vi "Find Setpoint.vi"(8 "error in (no error)":errorcluster, 11 "Settings in":T1 {"Processing Settings"."Test Parameters"."Allowed Tolerance (%) FS" format="%#_4g"; "Acq Settings"."Config Settings"."Simulated Sensor Injection" scale=0.0..100.0}) -> (0 "error out":errorcluster, 3 "Settings out":T1 {"Processing Settings"."Test Parameters"."Allowed Tolerance (%) FS" format="%#_4g"; "Acq Settings"."Config Settings"."Simulated Sensor Injection" scale=0.0..100.0})   [LabVIEW 2026]
uses:
  controls/UI/Settings Cluster.ctl
  controls/UI/Acq Settings.ctl
  Acquisition/Instrument Specifications Configuration.ctl
  Acquisition/Instrument Specifications Cluster Configuration.ctl
  controls/UI/Measurement Role.ctl
  controls/UI/Config Settings.ctl
  Processing/Processing Settings.ctl
  controls/Messaging Payloads/Sensor CoreData.ctl
  controls/Messaging Payloads/Sensor CoreData Cluster.ctl
  controls/UI/Units Enum.ctl
  controls/UI/Signal Enum.ctl
  Processing/Test Parameters.ctl
  Processing/Test Parameters Cluster.ctl
  controls/UI/Test Sequence Context.ctl
  controls/UI/Test Sequence Context Cluster.ctl
  controls/UI/Direction.ctl
  controls/UI/Session Identfiers.ctl
  controls/UI/Test Sequence Settings.ctl
  controls/UI/Test Sequence State.ctl
  controls/UI/Test Sequence Enum.ctl
  controls/Controller/Stimulus Settings.ctl
  controls/Controller/Stimulus Outputs.ctl
  controls/Controller/Stimulus Output.ctl
  controls/Controller/Controller Core Data.ctl
  controls/Controller/Stimulus Output Configuration.ctl
  controls/Controller/Stimulus Role.ctl
  Settings/Settings.lvlib
  Acquisition/Acquisition.lvlib
  Processing/Processing_Engine.lvlib
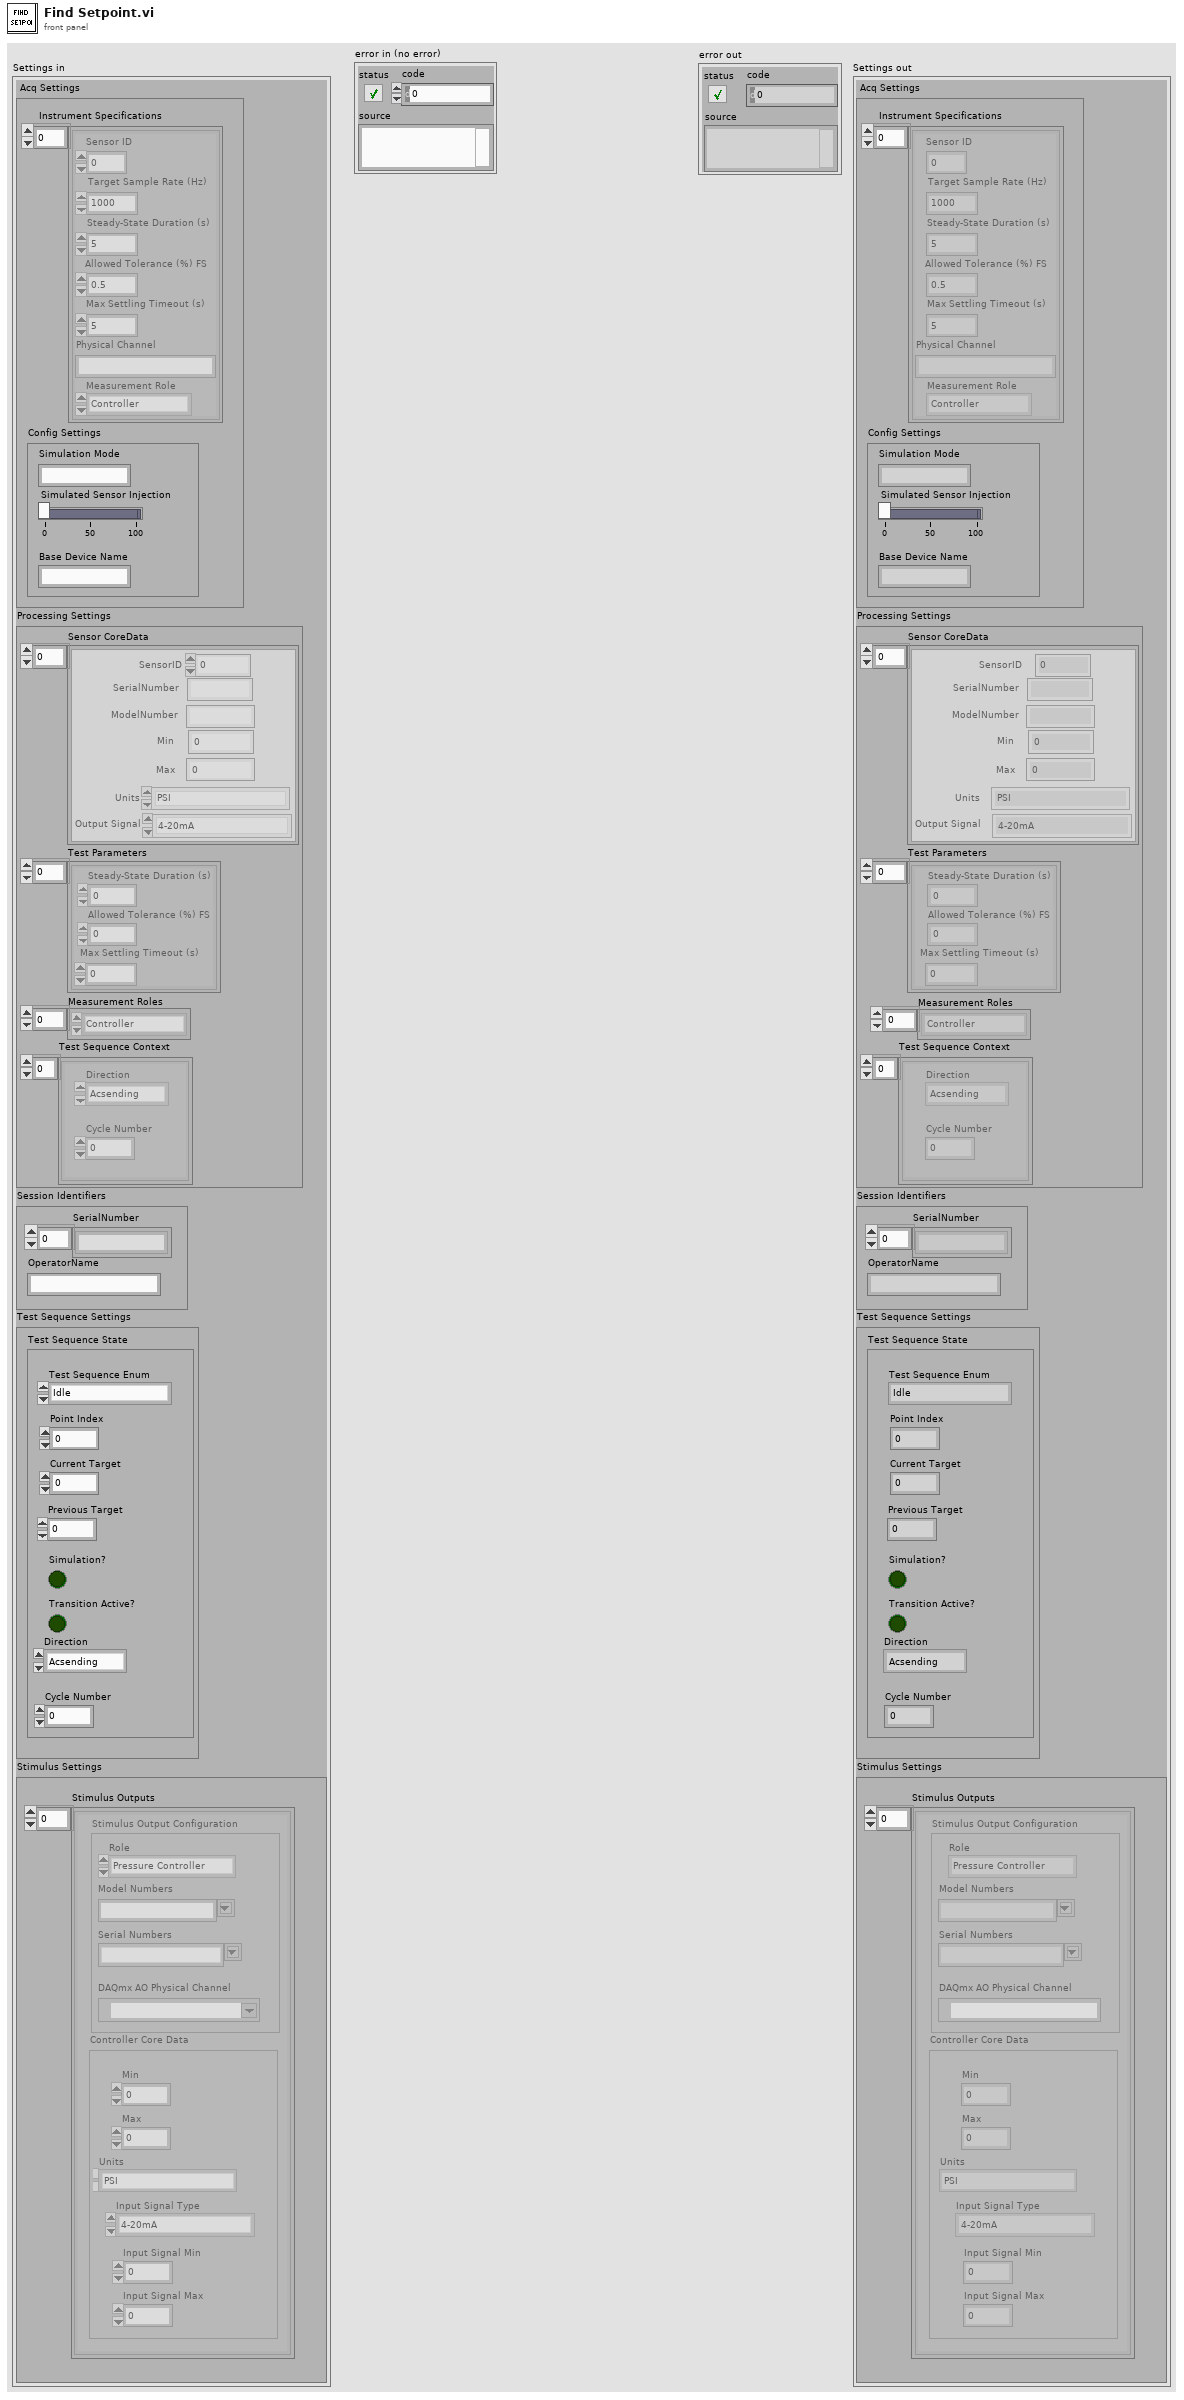
[diagram p1: front panel]
types:
  T1 = typedef "Settings Cluster.ctl" = cluster{"Acq Settings":T2, "Processing Settings":T7, "Session Identifiers":T17, "Test Sequence Settings":T18, "Stimulus Settings":T21}
  T2 = typedef "Acq Settings.ctl" = cluster{"Instrument Specifications":T3, "Config Settings":T6}
  T3 = typedef "Acquisition.lvlib/Instrument Specifications Configuration.ctl" = T4[]
  T4 = typedef "Acquisition.lvlib/Instrument Specifications Cluster Configuration.ctl" = cluster{"Sensor ID":i32, "Target Sample Rate (Hz)":dbl, "Steady-State Duration (s)":i32, "Allowed Tolerance (%) FS":dbl, "Max Settling Timeout (s)":i32, "Physical Channel":string, "Measurement Role":T5}
  T5 = typedef "Settings.lvlib/Measurement Role.ctl" = enum16{"Controller", "Reference", "UUT", "Disable", "All"}
  T6 = typedef "Config Settings.ctl" = cluster{"Simulated Sensor Injection":dbl, "Base Device Name":string, "Simulation Mode":string}
  T7 = typedef "Processing_Engine.lvlib/Processing Settings.ctl" = cluster{"Sensor CoreData":T8, "Test Parameters":T12, "Measurement Roles":T5[], "Test Sequence Context":T14}
  T8 = typedef "Sensor CoreData.ctl" = T9[]
  T9 = typedef "Settings.lvlib/Sensor CoreData Cluster.ctl" = cluster{"SerialNumber":string, "ModelNumber":string, "Min":dbl, "Max":dbl, "Units":T10, "Output Signal":T11, "SensorID":i32}
  T10 = typedef "Units Enum.ctl" = enum16{"PSI", "Deg C", "kPa", "GPM"}
  T11 = typedef "Signal Enum.ctl" = enum16{"4-20mA", "0-10V", "Thermocouple Type K"}
  T12 = typedef "Processing_Engine.lvlib/Test Parameters.ctl" = T13[]
  T13 = typedef "Settings.lvlib/Test Parameters Cluster.ctl" = cluster{"Steady-State Duration (s)":i32, "Allowed Tolerance (%) FS":dbl, "Max Settling Timeout (s)":i32}
  T14 = typedef "Settings.lvlib/Test Sequence Context.ctl" = T15[]
  T15 = typedef "Settings.lvlib/Test Sequence Context Cluster.ctl" = cluster{"Direction":T16, "Cycle Number":i32}
  T16 = typedef "Settings.lvlib/Direction.ctl" = enum16{"Acsending", "Descending"}
  T17 = typedef "Session Identfiers.ctl" = cluster{"SerialNumber":string[], "OperatorName":string}
  T18 = typedef "Test Sequence Settings.ctl" = cluster{"Test Sequence State":T19}
  T19 = typedef "Settings.lvlib/Test Sequence State.ctl" = cluster{"Test Sequence Enum":T20, "Point Index":i32, "Current Target":dbl, "Previous Target":dbl, "Simulation?":bool, "Direction":T16, "Transition Active?":bool, "Cycle Number":i32}
  T20 = typedef "Test Sequence Enum.ctl" = enum16{"Idle", "Start Point", "Point Complete", "Test Complete", "Abort Test", "Reset"}
  T21 = typedef "Settings.lvlib/Stimulus Settings.ctl" = cluster{"Stimulus Outputs":T22}
  T22 = typedef "Settings.lvlib/Stimulus Outputs.ctl" = T23[]
  T23 = typedef "Settings.lvlib/Stimulus Output.ctl" = cluster{"Controller Core Data":T24, "Stimulus Output Configuration":T25}
  T24 = typedef "Settings.lvlib/Controller Core Data.ctl" = cluster{"Min":dbl, "Max":dbl, "Units":T10, "Input Signal Type":T11, "Input Signal Min":dbl, "Input Signal Max":dbl}
  T25 = typedef "Settings.lvlib/Stimulus Output Configuration.ctl" = cluster{"DAQmx AO Physical Channel":tag, "Role":T26, "Model Numbers":string, "Serial Numbers":string}
  T26 = typedef "Stimulus Role.ctl" = enum16{"Pressure Controller", "Temperature Controller"}
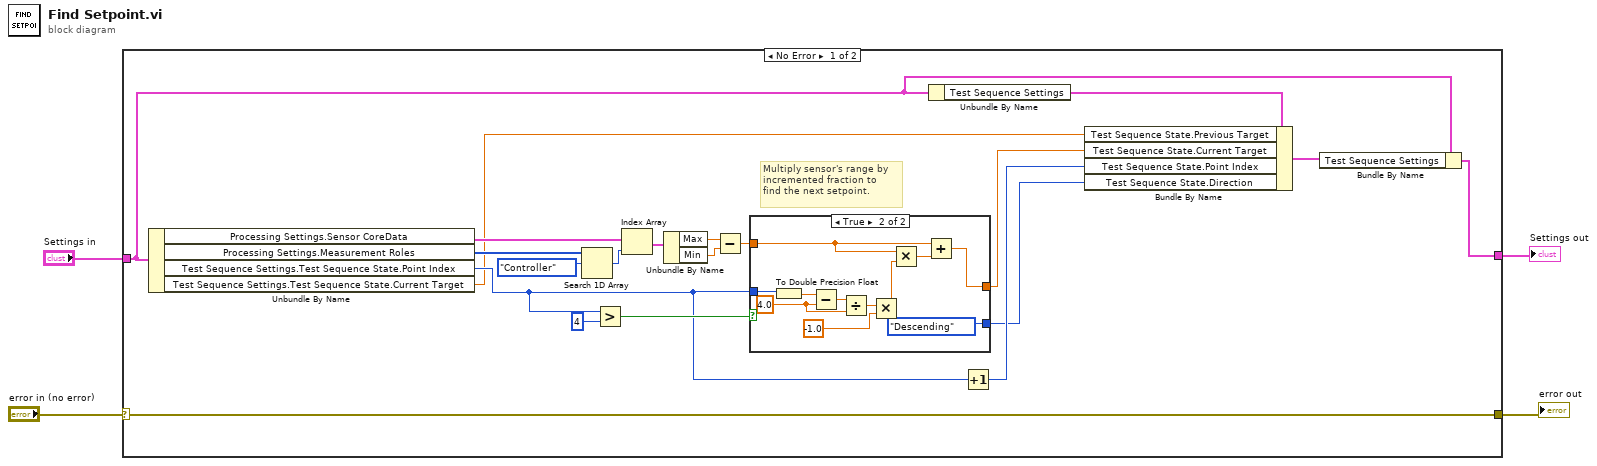
[diagram p0: block diagram]
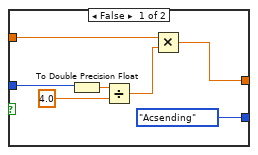
[diagram p2: hidden frame]
diagram:
  n1 = case shown="No Error" "error in (no error)" {
    selector: "error in (no error)" -> [w17 w44]
    tunnel: "Settings in" -> [w7 w43]
    tunnel: [w17 w44] -> w2
    tunnel: [w5 w43] -> w1
    frame No Error {
      # "Multiply sensor's range by\nincremented fraction to\nfind the next setpoint."
      n2 = Unbundle By Name(w7) -> ("Processing Settings.Sensor CoreData"=w20:T8, "Processing Settings.Measurement Roles"=w24:T5[], "Test Sequence Settings.Test Sequence State.Point Index"=w13:i32, "Test Sequence Settings.Test Sequence State.Current Target"=w12:dbl)
      n3 = Search 1D Array(1D array=w24, element=Measurement_Role."Controller") -> (index of element=w22:i32)  [unwired: 1 in]
      n4 = Greater?(x=w13, y=4) -> (0:w15:bool)
      n5 = Index Array(array=w20, index=w22) -> (element=w21:T9)
      n6 = Unbundle By Name(w21) -> ("Max"=w19:dbl, "Min"=w18:dbl)
      n7 = Subtract(x=w19, y=w18) -> (x-y=w14:dbl)
      n8 = case shown="True" w15 {
        tunnel: w13 -> [w29 w42]
        tunnel: w14 -> [w28 w34]
        tunnel: [w26 w33] -> w11
        tunnel: [Direction."Acsending" ("Direction") Direction."Descending" ("Direction")] -> w9
        frame False {
          n9 = To Double Precision Float(number=w29) -> (double precision float=w30:dbl)
          n10 = Divide(x=w30, y=4.0 ("number")) -> (x/y=w27:dbl)
          n11 = Multiply(x=w28, y=w27) -> (x*y=w26:dbl)
        }
        frame True {
          w38 = 4.0 ("number")
          n12 = To Double Precision Float(number=w42) -> (double precision float=w41:dbl)
          n13 = Subtract(x=w41, y=w38) -> (x-y=w39:dbl)
          n14 = Divide(x=w39, y=w38) -> (x/y=w37:dbl)
          n15 = Multiply(x=w37, y=-1.0 ("number")) -> (x*y=w36:dbl)
          n16 = Multiply(x=w34, y=w36) -> (x*y=w35:dbl)
          n17 = Add(x=w34, y=w35) -> (x+y=w33:dbl)
        }
      }
      n18 = Unbundle By Name(w7) -> ("Test Sequence Settings"=w8:T18)
      n19 = Increment(x=w13) -> (x+1=w10:i32)
      n20 = Bundle By Name(cluster=w8, "Test Sequence State.Previous Target"=w12, "Test Sequence State.Current Target"=w11, "Test Sequence State.Point Index"=w10, "Test Sequence State.Direction"=w9) -> (w6:T18)
      n21 = Bundle By Name(cluster=w7, "Test Sequence Settings"=w6) -> (w5:T1)
    }
    frame Error {
    }
  }
  "error out" <- w2
  "Settings out" <- w1
